vi "update tomo.vi"(8 "error in (no error)":errorcluster, 11 "Autofocus in":refnum<class "Autofocus.lvclass">) -> (0 "error out":errorcluster, 3 "Autofocus out":refnum<class "Autofocus.lvclass">)   [LabVIEW 2012, in "Autofocus.lvclass"]
uses:
  Autofocus.lvclass
  <vilib>/Distrio/Murmex/Murmex/update_cluster.ctl
  Autofocus.lvclass/Autofocus.ctl
  <vilib>/Distrio/Murmex/Murmex/Murmex.lvclass
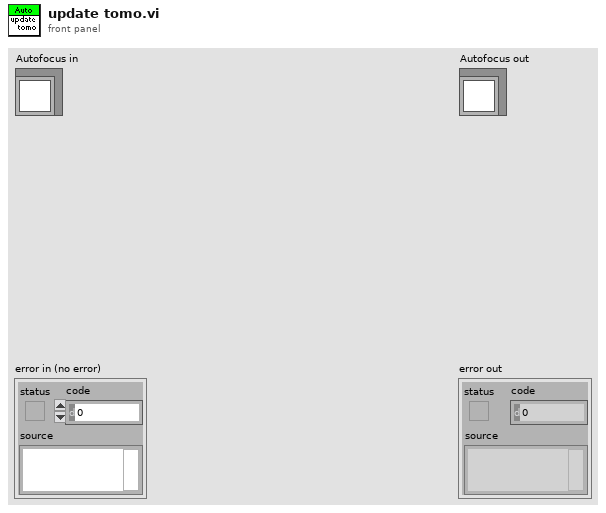
[diagram p1: front panel]
types:
  T1 = typedef "Murmex.lvlib/Murmex.lvclass/update_cluster.ctl" = cluster{"target ID":string, "key chains":string[], "values":variant[]}
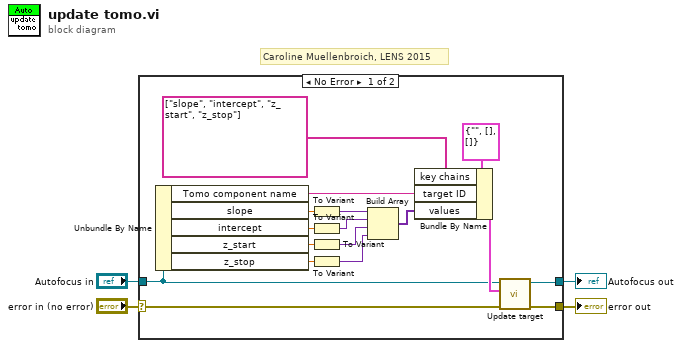
[diagram p0: block diagram]
diagram:
  # "Caroline Muellenbroich, LENS 2015"
  n1 = case shown="No Error" "error in (no error)" {
    selector: "error in (no error)" -> [w15 w23]
    tunnel: [w5 w23] -> w3
    tunnel: [w6 w22] -> w1
    tunnel: "Autofocus in" -> [w14 w22]
    frame No Error {
      n2 = Unbundle By Name(w14) -> ("Tomo component name"=w21:string, "slope"=w10:dbl, "intercept"=w9:dbl, "z_start"=w8:dbl, "z_stop"=w7:dbl)
      n3 = To Variant(anything=w10) -> (Variant=w17:variant)
      n4 = To Variant(anything=w9) -> (Variant=w13:variant)
      n5 = To Variant(anything=w8) -> (Variant=w12:variant)
      n6 = To Variant(anything=w7) -> (Variant=w11:variant)
      n7 = Build Array(w17, w13, w12, w11) -> (w18:variant[])
      n8 = Bundle By Name(cluster=T1 {"target ID"="", "key chains"=[], "values"=[]} ("update cluster"), "key chains"=string[] ["slope", "intercept", "z_start", "z_stop"], "target ID"=w21, "values"=w18) -> (w19:T1)
      n9 = call <vilib>:"Update target.vi"("error in (no error)"=w15, "update cluster"=w19, "MurmexBase in"=w14) -> ("error out"=w5:errorcluster, "MurmexBase out"=w6:refnum<class "Autofocus.lvclass">)  [unwired: 7 in]
    }
    frame Error {
    }
  }
  "error out" <- w3
  "Autofocus out" <- w1
